vi "Handle.vi"(11 "Dev Actor in":refnum<class "Dev Actor.lvclass">) -> (2 "Destroy?":bool, 3 "Dev Actor out":refnum<class "Dev Actor.lvclass">)   [LabVIEW 2021, in "Dev Actor.lvlib" / "Dev Actor.lvclass"]
uses:
  Dev Actor.lvclass
  Dev Actor.lvclass/Dev Actor.ctl
  Actor/Queue Actor/Queue Actor.lvclass
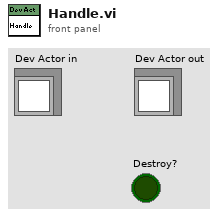
[diagram p1: front panel]
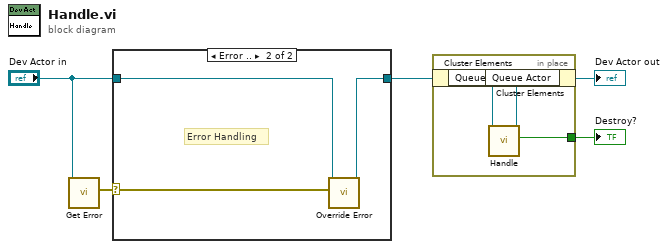
[diagram p0: block diagram]
diagram:
  n1 = call-dynamic "Get Error.vi"("Dev Actor in"="Dev Actor in") -> ("Error"=w1:errorcluster)  [unwired: 10 in]
  n2 = case shown="Error .." w1 {
    selector: w1 -> [_ w7]
    tunnel: "Dev Actor in" -> [w6 w9]
    tunnel: [w6 w8] -> w4
    frame No Error {
    }
    frame Error {
      # "Error Handling"
      n3 = call-dynamic "Override Error.vi"("Error"=w7, "Dev Actor in"=w9) -> ("Dev Actor out"=w8:refnum<class "Dev Actor.lvclass">)  [unwired: 9 in]
    }
  }
  n4 = in-place {
    in-place-border: [w10] -> w3
    n5 = in-place-cluster #1(w4) -> ("Queue Actor"=w12:refnum<class "Queue Actor.lvclass">)
    n6 = call-dynamic "Handle.vi"("Actor in"=w12) -> ("Destroy?"=w10:bool, "Actor out"=w11:refnum<class "Queue Actor.lvclass">)  [unwired: 9 in]
    n7 = in-place-cluster #1("Queue Actor"=w11) -> (→"Dev Actor out":refnum<class "Dev Actor.lvclass">)
  }
  "Destroy?" <- w3
